vi "Get fixed_coords.vi"(11 "raw data in":u8[](array[numeric])) -> (1 "valid":bool=TRUE, 3 "eu data out":dbl[](array[numeric]))   [LabVIEW 2019, in "HLA Data Conversion.lvlib"]
uses:
  HLA Data Conversion.lvlib
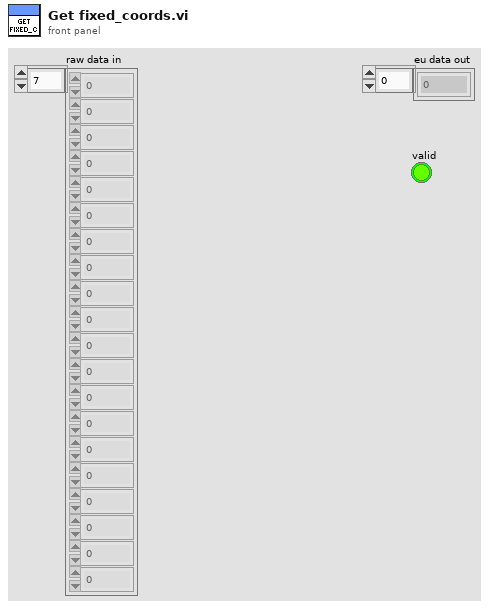
[diagram p1: front panel]
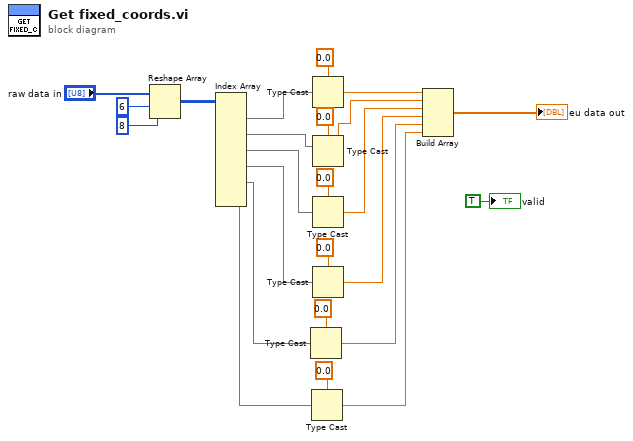
[diagram p0: block diagram]
diagram:
  n1 = Reshape Array("raw data in", 6 ("dimension size"), 8 ("dimension size")) -> (w21:u8[][])
  n2 = Index Array(array=w21) -> (element #1=w20:u8[], element #2=w14:u8[], element #3=w8:u8[], element #4=w7:u8[], element #5=w6:u8[], element #6=w5:u8[])  [unwired: 12 in]
  n3 = Type Cast(type=0.0 ("world.location.x"), x=w6) -> (*(type *) &x=w10:dbl)
  n4 = Type Cast(type=0.0 ("world.location.x"), x=w5) -> (*(type *) &x=w9:dbl)
  n5 = Type Cast(type=0.0 ("world.location.x"), x=w20) -> (*(type *) &x=w22:dbl)
  n6 = Type Cast(type=0.0 ("world.location.x"), x=w14) -> (*(type *) &x=w13:dbl)
  n7 = Type Cast(type=0.0 ("world.location.x"), x=w8) -> (*(type *) &x=w12:dbl)
  n8 = Type Cast(type=0.0 ("world.location.x"), x=w7) -> (*(type *) &x=w11:dbl)
  n9 = Build Array(w22, w13, w12, w11, w10, w9) -> (→"eu data out":dbl[])
  "valid" <- TRUE
